vi "AcquireImage test.vi"() -> ()   [LabVIEW 2009]
uses:
  Camera.lvlib
  ImageAnalysis.lvlib
panel:
  out "Objects bottom cords 2":cluster{"Cord":cluster{"X":dbl, "Y":dbl}[]}[](array[cluster])
  out "Objects bottom cords":cluster{"Cord":cluster{"X":dbl, "Y":dbl}[]}[](array[cluster])
  out "Numeric":i32
  in  "stop":bool
  out "Image":T1(plugin-control)
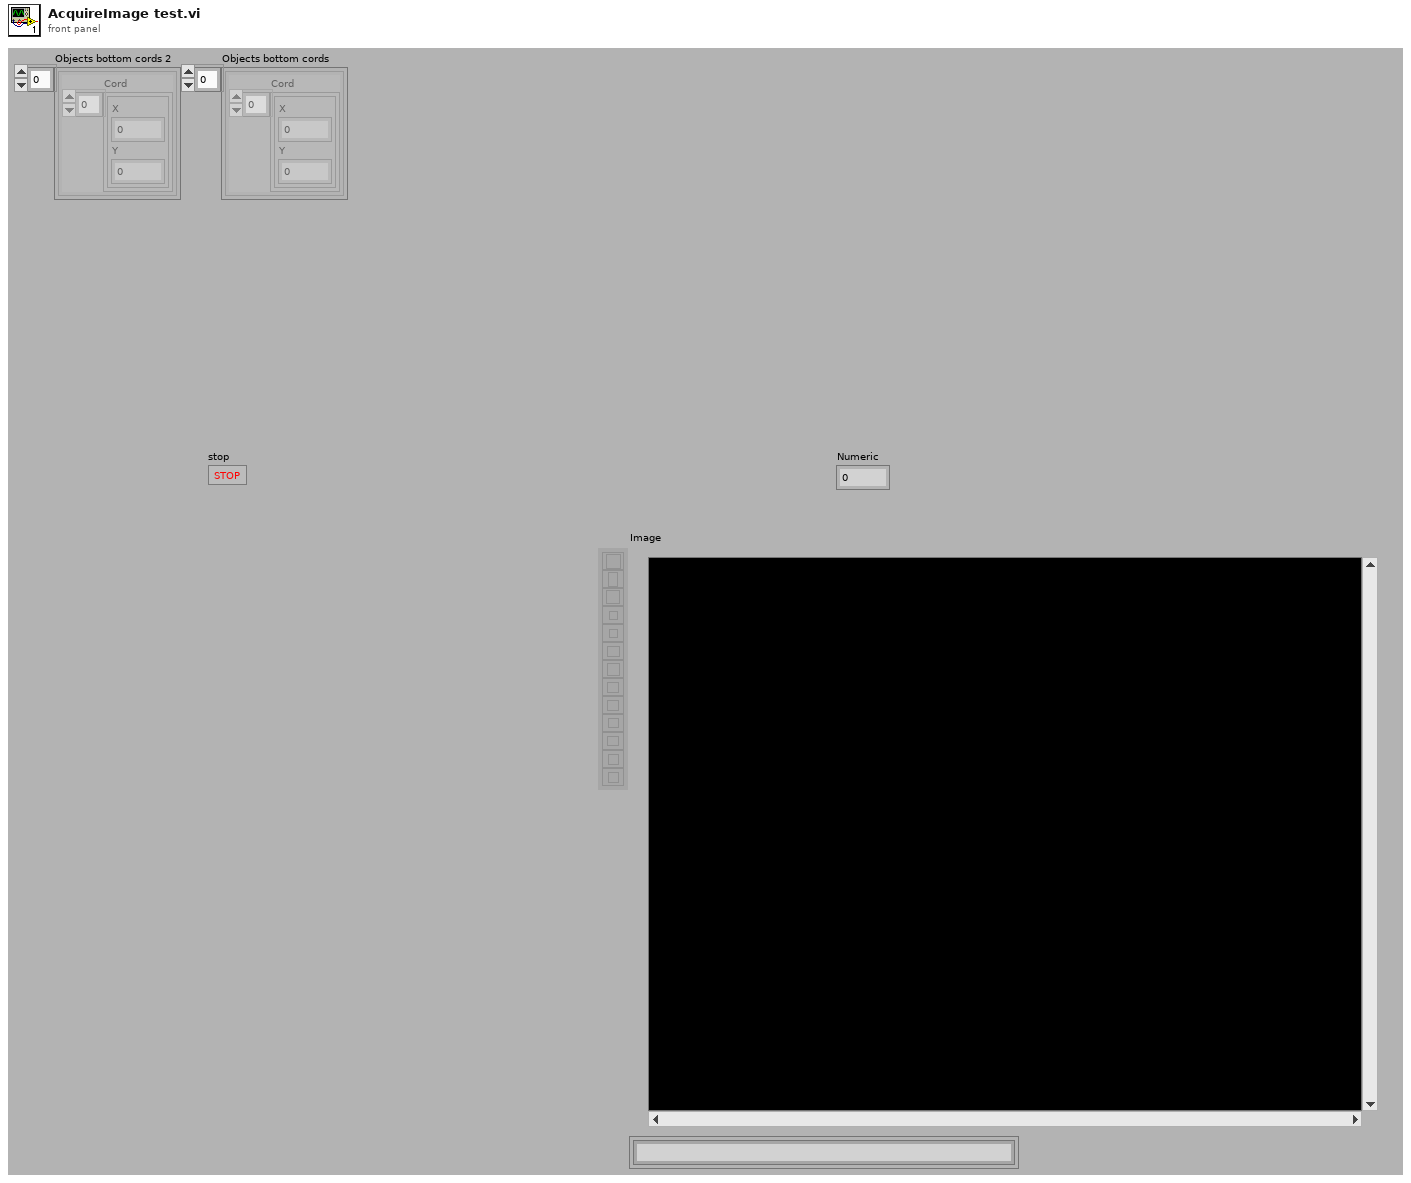
[diagram p1: front panel]
types:
  T1 = typedef "IMAQ Image.ctl" = refnum<image>
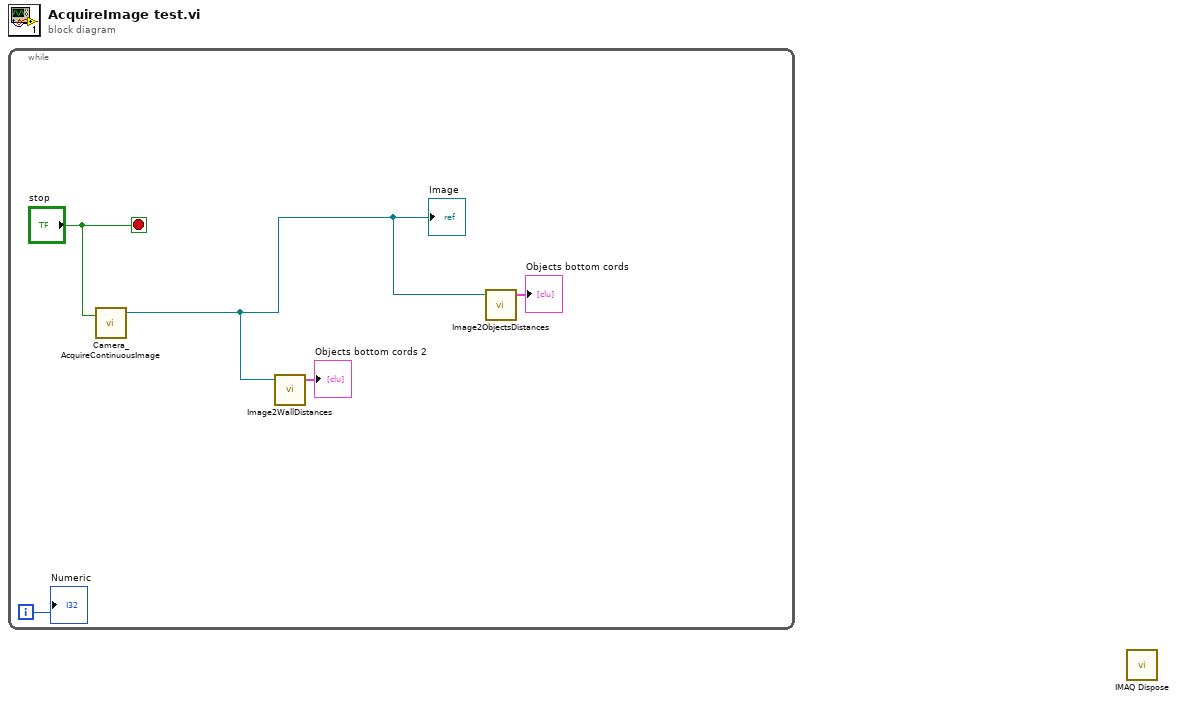
[diagram p0: block diagram]
diagram:
  n1 = while {
    i -> [w4]
    stop <- "stop" stop-if-true
    n2 = call "Camera_AcquireContinuousImage.vi"("Stop (F)"="stop") -> ("Image Out"=w1:T1)  [unwired: 1 in, 2 out]
    "Image" <- w1
    n3 = call "Image2WallDistances.vi"("Image Src"=w1) -> ("Objects bottom cords"=→"Objects bottom cords 2":cluster{"Cord":cluster{"X":dbl, "Y":dbl}[]}[])  [unwired: 3 in, 1 out]
    n4 = call "Image2ObjectsDistances.vi"("Image Src"=w1) -> ("Objects bottom cords"=→"Objects bottom cords":cluster{"Cord":cluster{"X":dbl, "Y":dbl}[]}[])  [unwired: 3 in, 1 out]
    "Numeric" <- w4
  }
  n5 = call "IMAQ Dispose"() -> ()  [unwired: 6 in, 1 out]
